vi "tanh.vi"(1 "x":T1) -> (0 "y":T1)   [LabVIEW 2020]
uses:
  <vilib>/Analysis/Matrix/Datatypes/RealMatrix.ctl
  <vilib>/Analysis/Matrix/Numeric/Conversions/Array To Matrix - RA.vi
  <vilib>/Analysis/Matrix/NI_Matrix.lvlib
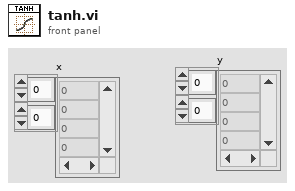
[diagram p1: front panel]
types:
  T1 = typedef "NI_Matrix.lvlib/RealMatrix.ctl" = dbl[][]
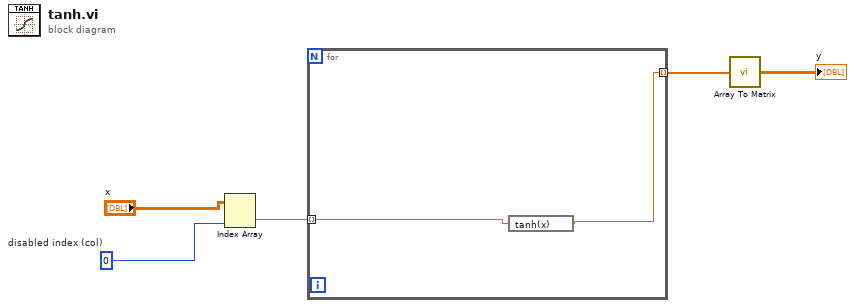
[diagram p0: block diagram]
diagram:
  w1 = 0  # disabled index (col)
  n1 = Index Array(array="x", index (col)=w1) -> (element=w5:dbl[])  [unwired: 1 in]
  n2 = for {
    tunnel: w5 -> [w7] mode=indexing
    tunnel: [w6] -> w4 mode=indexing
    n3 = expression code="tanh(x)"(w7) -> (w6:dbl)
  }
  n4 = call-poly <vilib>:"Array To Matrix.vi"("Real 1D Array"=w4) -> ("Real Matrix (Column Vector)"=→"y":T1)
